vi "SaveVexesTdm.vi"(2 "error in":errorcluster, 3 "VExes":dbl, 4 "Vbreak":dbl, 5 "storage refnum (file)":refnum<k20>) -> (0 "error out":errorcluster, 1 "storage refnum (file) 3":refnum<k20>)   [LabVIEW 2014]
uses:
  <vilib>/Platform/storage/Storage.llb/usiSequenceRepresentation.ctl
  <vilib>/Platform/storage/Storage.llb/usiOverwriteOptions.ctl
  <vilib>/Platform/storage/lvStorage.llb/_createOrGetByNameExplicitChildObject.vi
  <vilib>/Platform/storage/Storage.llb/__savePropString.vi
  <vilib>/Platform/storage/lvStorage.llb/xStorage/xStorageSupp/ErrorOut.vi
  <vilib>/Platform/storage/lvStorage.llb/__saveFloat64Channel.vi
  <vilib>/Platform/storage/lvStorage.llb/xStorage/Write Data/Write Data.xnode
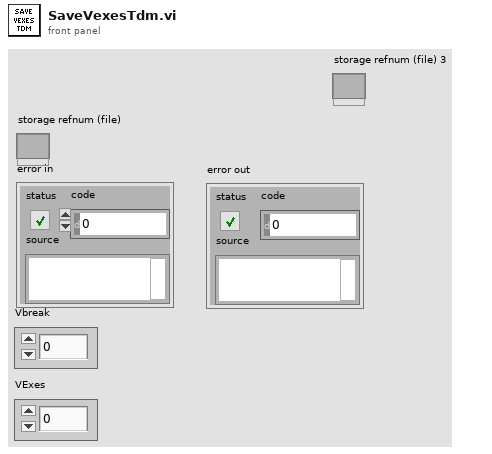
[diagram p1: front panel]
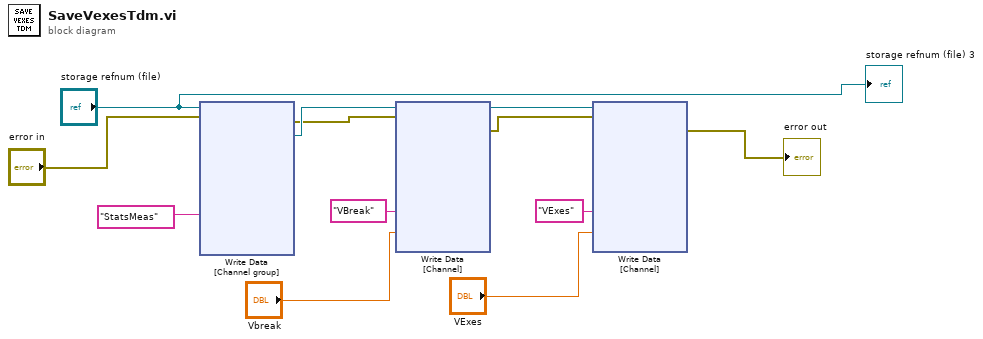
[diagram p0: block diagram]
diagram:
  n1 = xnode "Write Data\n[Channel group]"("Name"="StatsMeas", "storage refnum (file)"="storage refnum (file)", "error in"="error in") -> ("error out"=w11:errorcluster, "storage refnum (channel group)"=w12:refnum<k20>)  [unwired: 1 in, 1 out]
  n2 = xnode "Write Data\n[Channel]"("Name"="VBreak", "Signal"="Vbreak", "storage refnum (channel group)"=w12, "error in"=w11) -> ("storage refnum (channel group) out"=w10:refnum<k20>, "error out"=w9:errorcluster)  [unwired: 2 in, 1 out]
  n3 = xnode "Write Data\n[Channel]"("Name"="VExes", "Signal"="VExes", "storage refnum (channel group)"=w10, "error in"=w9) -> ("error out"=→"error out":errorcluster)  [unwired: 2 in, 2 out]
  "storage refnum (file) 3" <- "storage refnum (file)"
